vi "FeedbackDecode_GetAllControlReferences.vi"(3 "error in":errorcluster, 5 "RefArray":refnum<vi>[](array[refnum])) -> (0 "error out":errorcluster, 1 "KeyFocus":bool, 2 "controls[]":refnum<vi>[](array[refnum]))   [LabVIEW 2016]
doc: "The Get All Control References VI recursively determines control references for all objects on the front panel of another VI. This VI takes a front panel reference input and returns an array of references to all controls on that front panel. This VI returns references to all elements of a cluster, including elements in embedded clusters. This VI also returns the element types of arrays embedded in cluster elements."
panel:
  in  "target class 3":refnum<vi>
  in  "target class 2":refnum<vi>
  in  "target class":refnum<vi>
  # "Select Help»Show Context Help and move the cursor over the VI icon to display help for this VI."
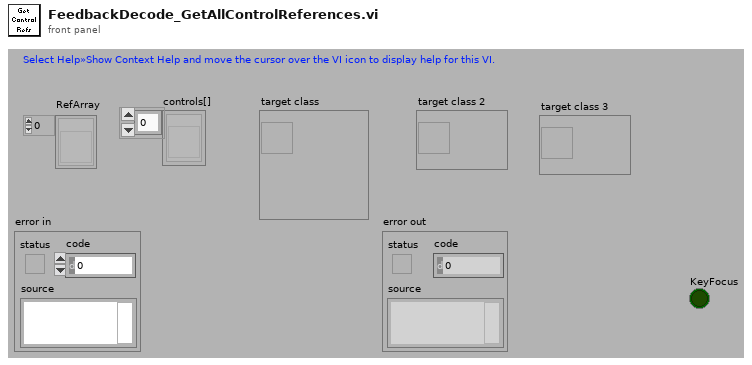
[diagram p1: front panel]
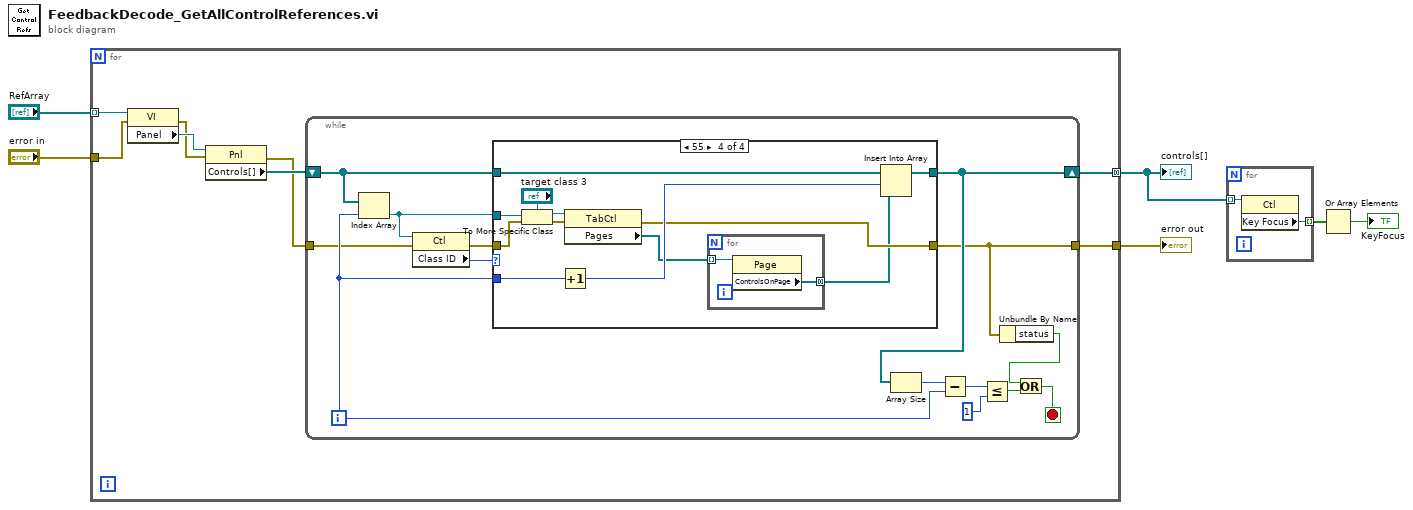
[diagram p0: block diagram]
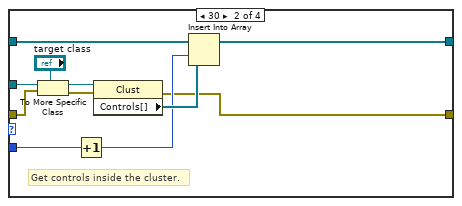
[diagram p3: hidden frame]
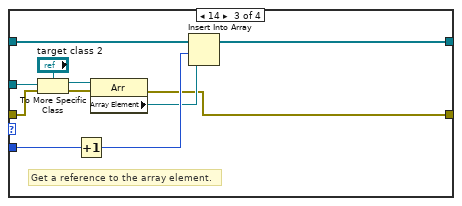
[diagram p4: hidden frame]
diagram:
  n1 = for {
    tunnel: [w12] -> w6
    tunnel: [w10] -> w5 mode=concatenating
    tunnel: "RefArray" -> [w9] mode=indexing
    tunnel: "error in" -> [w8]
    n2 = property class="VI"(reference=w9, error in=w8) -> (error out=w7:errorcluster, "Panel"=w11:refnum<vi>)  [unwired: 1 out]
    n3 = property class="Pnl"(reference=w11, error in=w7) -> (error out=w13:errorcluster, "Controls[]"=w14:refnum<vi>[])  [unwired: 1 out]
    n4 = while {
      shift-right: [w19] -> w10
      shift-left: w14 -> [w20]
      tunnel: w13 -> [w18]
      tunnel: [w15] -> w12
      i -> [w25]
      stop <- w23 stop-if-true
      n5 = Index Array(array=w20, index=w25) -> (element=w21:refnum<vi>)
      n6 = property class="Ctl"(reference=w21, error in=w18) -> (error out=w17:errorcluster, "Class ID"=w22:u32)  [unwired: 1 out]
      n7 = case shown="55" w22 {
        tunnel: w21 -> [_ w41 w52 w64]
        tunnel: w20 -> [w30 w38 w49 w61]
        tunnel: w25 -> [_ w37 w48 w60]
        tunnel: [w30 w35 w47 w59] -> w19
        tunnel: w17 -> [w29 w33 w44 w57]
        tunnel: [w29 w31 w42 w55] -> w15
        frame 0, Default {
        }
        frame 30 {
          # "Get controls inside the cluster."
          n8 = To More Specific Class(target class="target class", reference=w41, error in=w33) -> (specific class reference=w40:refnum<vi>, error out=w32:errorcluster)
          n9 = Increment(x=w37) -> (x+1=w34:i32)
          n10 = property class="Clust"(reference=w40, error in=w32) -> (error out=w31:errorcluster, "Controls[]"=w36:refnum<vi>[])  [unwired: 1 out]
          n11 = Insert Into Array(array=w38, index=w34, new element=w36) -> (w35:refnum<vi>[])
        }
        frame 14 {
          # "Get a reference to the array element."
          n12 = To More Specific Class(target class="target class 2", reference=w52, error in=w44) -> (specific class reference=w51:refnum<vi>, error out=w43:errorcluster)
          n13 = Increment(x=w48) -> (x+1=w46:i32)
          n14 = property class="Arr"(reference=w51, error in=w43) -> (error out=w42:errorcluster, "Array Element"=w45:refnum<vi>)  [unwired: 1 out]
          n15 = Insert Into Array(array=w49, index=w46, new element=w45) -> (w47:refnum<vi>[])
        }
        frame 55 {
          n16 = To More Specific Class(target class="target class 3", reference=w64, error in=w57) -> (specific class reference=w63:refnum<vi>, error out=w56:errorcluster)
          n17 = Increment(x=w60) -> (x+1=w58:i32)
          n18 = property class="TabCtl"(reference=w63, error in=w56) -> (error out=w55:errorcluster, "Pages"=w54:refnum<vi>[])  [unwired: 1 out]
          n19 = for {
            tunnel: w54 -> [w66] mode=indexing
            tunnel: [w65] -> w53 mode=concatenating
            n20 = property class="Page"(reference=w66) -> ("ControlsOnPage"=w65:refnum<vi>[])  [unwired: 1 in, 2 out]
          }
          n21 = Insert Into Array(array=w61, index=w58, new element=w53) -> (w59:refnum<vi>[])
        }
      }
      n22 = Array Size(array=w19) -> (size(s)=w28:i32)
      n23 = Subtract(x=w28, y=w25) -> (x-y=w27:i32)
      n24 = Less Or Equal?(x=w27, y=1) -> (x <= y?=w24:bool)
      n25 = Unbundle By Name(w15) -> ("status"=w16:bool)
      n26 = Or(x=w16, y=w24) -> (x .or. y?=w23:bool)
    }
  }
  "controls[]" <- w5
  "error out" <- w6
  n27 = for {
    tunnel: w5 -> [w68] mode=indexing
    tunnel: [w67] -> w4 mode=indexing
    n28 = property class="Ctl"(reference=w68) -> ("Key Focus"=w67:bool)  [unwired: 1 in, 2 out]
  }
  n29 = Or Array Elements(Boolean array=w4) -> (logical OR=→"KeyFocus":bool)
